vi "ClusterToFlags.vi"(8 "error in":errorcluster, 10 "RoomNumFlags":T1={"Flag State"=[1, 3, 5, 7]}) -> (0 "error out":errorcluster, 2 "State":bool[](array[boolean]))   [LabVIEW 2015, in "DatabaseApi.lvlib"]
uses:
  LVClasses/Flags/ColorFlags.ctl
  LVClasses/Flags/Flags.lvclass/Flags.ctl
  DatabaseApi.lvlib
  LVClasses/Flags/Flags.lvclass
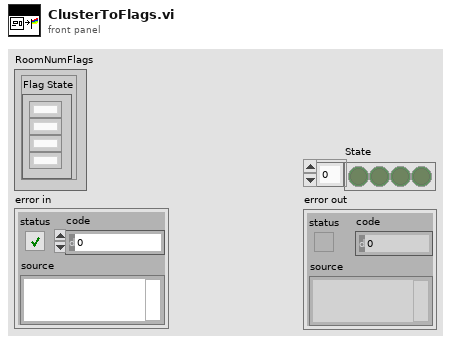
[diagram p1: front panel]
types:
  T1 = typedef "Flags.lvclass/ColorFlags.ctl" = cluster{"Flag State":u8[]}
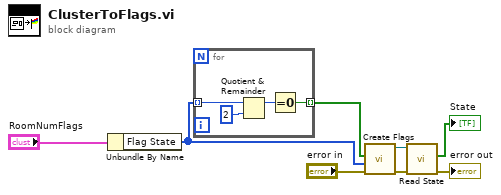
[diagram p0: block diagram]
diagram:
  n1 = Unbundle By Name("RoomNumFlags") -> ("Flag State"=w3:u8[])
  n2 = for {
    tunnel: w3 -> [w12] mode=indexing
    tunnel: [w9] -> w2 mode=indexing
    n3 = Quotient & Remainder(x=w12, y=u8 2) -> (x-y*floor(x/y)=w10:u8)  [unwired: 1 out]
    n4 = Equal To 0?(x=w10) -> (x = 0?=w9:bool)
  }
  n5 = call "Create Flags.vi"("error in"="error in", "Color"=w3, "State"=w2) -> ("error out"=w7:errorcluster, "reference out"=w6:refnum<class "Flags.lvclass">)  [unwired: 7 in]
  n6 = call "Read State.vi"("error in (no error)"=w7, "Flags in"=w6) -> ("error out"=→"error out":errorcluster, "State"=→"State":bool[])  [unwired: 7 in, 1 out]
